vi "Galvo+Histo.vi"() -> ()   [LabVIEW 2016]
uses:
  <vilib>/Utility/error.llb/DialogType.ctl
  <vilib>/DAQmx/write.llb/DAQmx Write (Analog 1D DBL NChan 1Samp).vi
  <vilib>/DAQmx/write.llb/DAQmx Write (Analog DBL 1Chan 1Samp).vi
  <vilib>/DAQmx/create/channels.llb/DAQmx Create Channel (AO-Voltage-Basic).vi
  <vilib>/DAQmx/miscellaneous.llb/DAQmx Fill In Error Info.vi
  HHLib64.dll
panel:
  in  "Run":bool
  in  "done":bool
  in  "Syncdiv":enum16{"1", "2", "4", "8"}(ring)
  in  "Binning":i32 min=0 max=10 step=1
  in  "Sync Level":i32=50 min=0 max=800 step=10
  in  "Ch1 Level":i32=50 min=0 max=800 step=10
  in  "Ch1 ZeroX":i32=10 min=0 max=20 step=1
  in  "Sync ZeroX":i32=10 min=0 max=20 step=1
  in  "Sync Offs":i32=-10000 min=-99999 max=99999 step=1
  in  "Ch1 Offs":i32 min=-99999 max=99999 step=1
  in  "Ch2 Level":i32=50 min=0 max=800 step=10
  in  "Ch2 ZeroX":i32=10 min=0 max=20 step=1
  in  "Ch2 Offs":i32 min=-99999 max=99999 step=1
  in  "Ch3 Level":i32=50 min=0 max=800 step=10
  in  "Ch3 ZeroX":i32=10 min=0 max=20 step=1
  in  "Ch3 Offs":i32 min=-99999 max=99999 step=1
  in  "Ch4 Offs":i32 min=-99999 max=99999 step=1
  in  "Ch4 Level":i32=50 min=0 max=800 step=10
  in  "Ch4 ZeroX":i32=10 min=0 max=20 step=1
  out "Resol / ps":dbl format="%.2f"
  in  "Ch8 ZeroX":i32=10 min=0 max=20 step=1
  in  "Ch8 Level":i32=50 min=0 max=800 step=10
  in  "Ch8 Offs":i32 min=-99999 max=99999 step=1
  in  "Ch7 Offs":i32 min=-99999 max=99999 step=1
  in  "Ch7 ZeroX":i32=10 min=0 max=20 step=1
  in  "Ch7 Level":i32=50 min=0 max=800 step=10
  in  "Ch5 Level":i32=50 min=0 max=800 step=10
  in  "Ch6 Level":i32=50 min=0 max=800 step=10
  in  "Ch5 ZeroX":i32=10 min=0 max=20 step=1
  in  "Ch6 ZeroX":i32=10 min=0 max=20 step=1
  in  "Ch5 Offs":i32 min=-99999 max=99999 step=1
  in  "Ch6 Offs":i32 min=-99999 max=99999 step=1
  out "Oveflow":bool
  out "Histogram":u32[][](graph)
  out "IntegralCount":i32[](array[numeric])
  in  "Acq.Time /ms":i32=1000 min=1 max=3600000 step=100
  out "Rate 4":i32(slide) scale=0.01..100000000.0 scale format="%.0e"
  out "Rate 3":i32(slide) scale=0.01..100000000.0 scale format="%.0e"
  out "Rate 2":i32(slide) scale=0.01..100000000.0 scale format="%.0e"
  out "Rate 1":i32(slide) scale=0.01..100000000.0 scale format="%.0e"
  out "Sync Rate":i32(slide) scale=0.01..100000000.0 scale format="%.0e"
  out "Rate 6":i32(slide) scale=0.01..100000000.0 scale format="%.0e"
  out "Rate 5":i32(slide) scale=0.01..100000000.0 scale format="%.0e"
  out "Rate 7":i32(slide) scale=0.01..100000000.0 scale format="%.0e"
  out "Rate 8":i32(slide) scale=0.01..100000000.0 scale format="%.0e"
  out "Warnings":string
  out "Serial Num.":string
  out "DeviceIndex":i32=-1
  out "DLL Version (must be 2.0)":string caption="DLL Version"
  out "Calibration Status":string
  out "Initialization Status":string
  in  "Hold/Scan":enum32{"Hold", "Radio Selection 2"}(radio)
  in  "Max Voltage":dbl=10.0
  in  "Min Voltage Voltage":dbl=-10.0
  in  "Set this opposite to one above":tag="Dev1/ao0"
  out "Current Voltage":dbl
  out "Next Voltage":dbl
  in  "Wait Time (ms)":dbl=100.0
  in  "Max Voltage 2":dbl=10.0
  in  "Min Voltage Voltage 2":dbl=-10.0
  in  "Scan in X: Set to ao1\nScan in Y: Set to ao0":tag="Dev1/ao0"
  out "Current Voltage 2":dbl
  out "Next Voltage 2":dbl
  in  "Wait Time (ms) 2":dbl=100.0
  in  "Voltage Step 2":dbl=0.1
  in  "Voltage Step":dbl=0.1
  in  "Physical Channel(s)":tag="Dev1/ao0"
  in  "Stop":bool
  in  "Output Voltage":dbl[](array[numeric])
  in  "Min Voltage":dbl=-10.0
  in  "Max Voltage 3":dbl=10.0
  in  "Physical Channel(s)  2":tag="Dev1/ao0"
  in  "Stop 2":bool
  in  "Output Voltage 2":dbl[](array[numeric])
  in  "Min Voltage 2":dbl=-10.0
  in  "Max Voltage 4":dbl=10.0
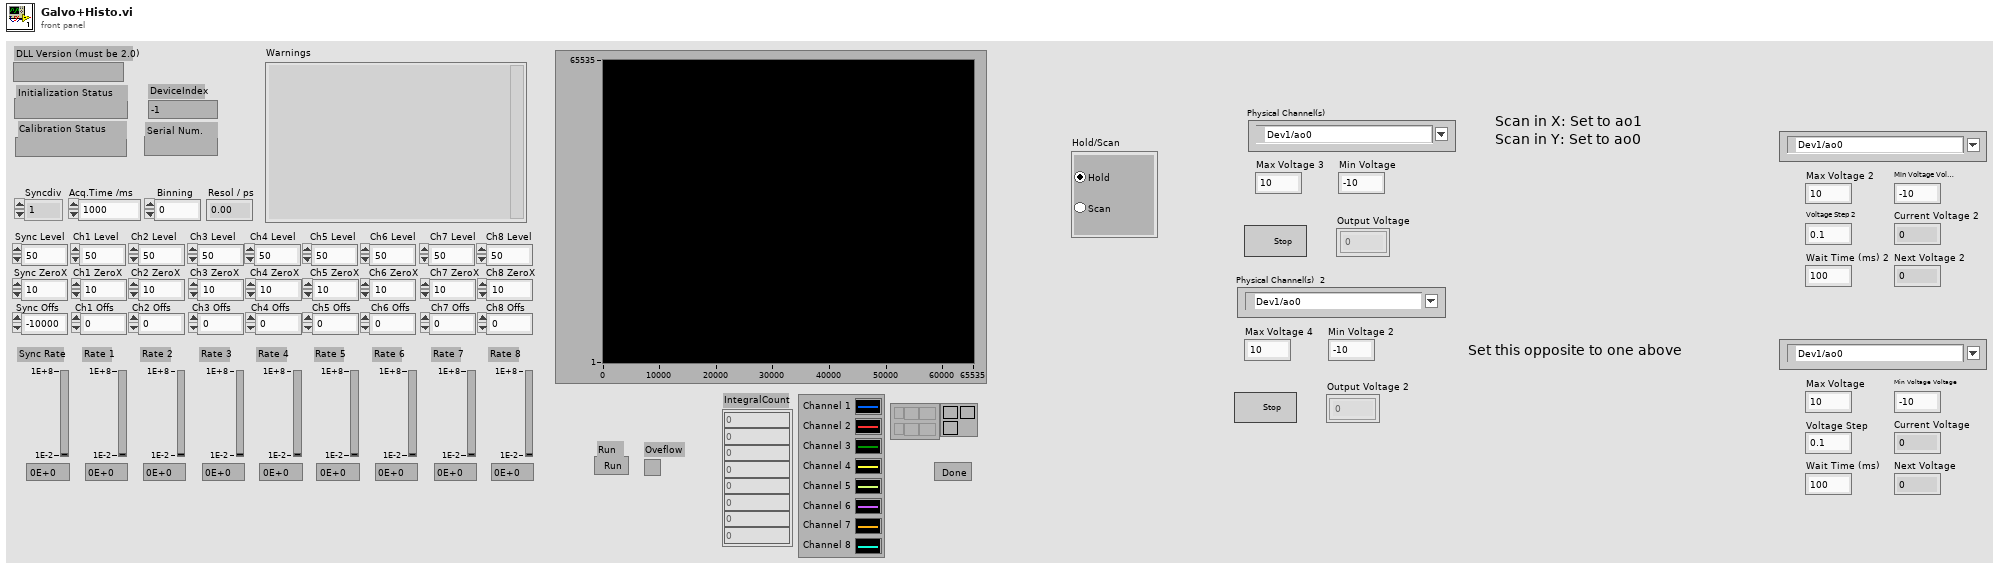
[diagram p1: front panel]
types:
  T1 = cluster{"rate":i32, "rate":i32, "rate":i32, "rate":i32, "rate":i32, "rate":i32, "rate":i32, "rate":i32}
  T2 = typedef "DialogType.ctl" = u16
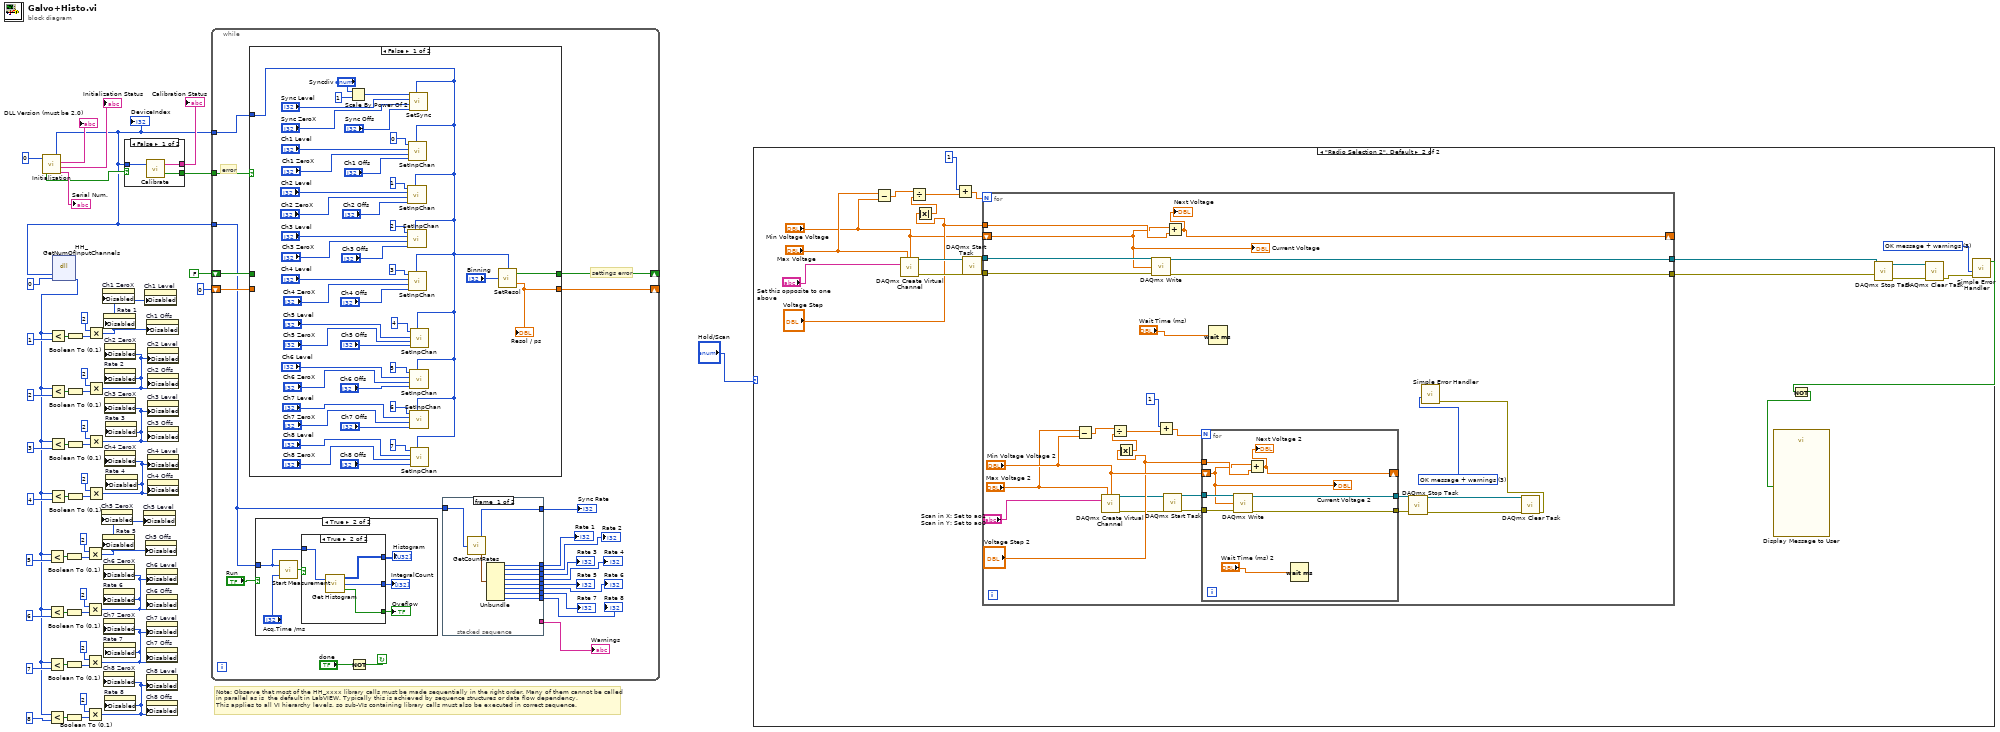
[diagram p0: block diagram]
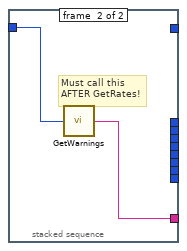
[diagram p2: hidden frame]
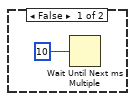
[diagram p3: hidden frame]
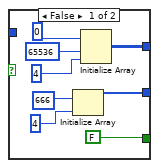
[diagram p4: hidden frame]
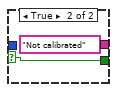
[diagram p6: hidden frame]
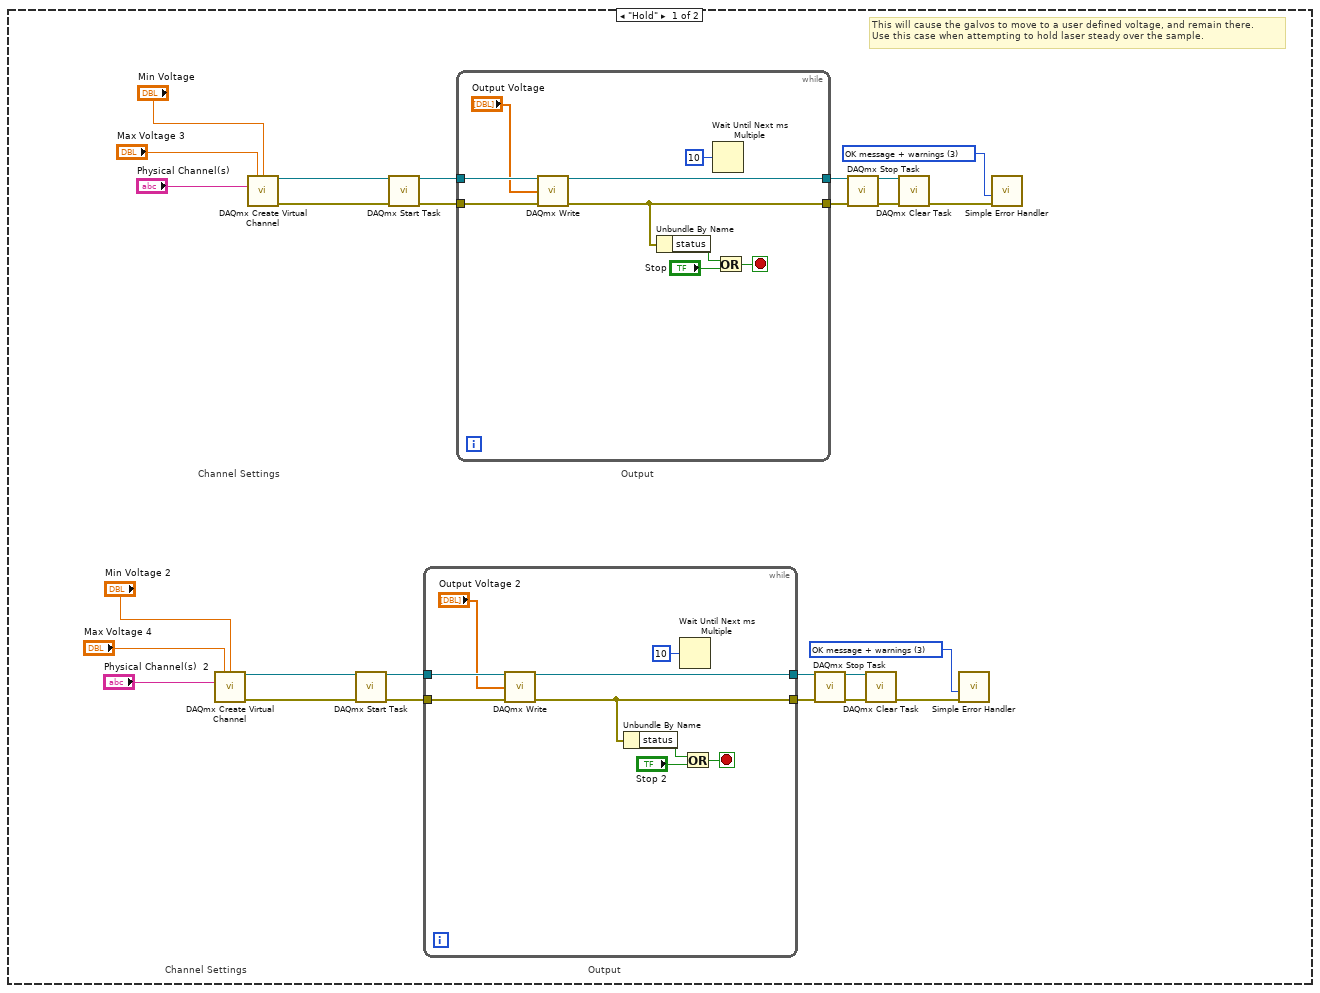
[diagram p7: hidden frame]
diagram:
  # "settings error"
  # "Note: Observe that most of the HH_xxxx library calls must be made sequentially in the right order. Many of them cannot be called \nin parallel as is  the default in LabVIEW. Typically this is achieved by sequence structures or data flow dependency. \nThis applies to all VI hierarchy levels, so sub-VIs containing library calls must also be executed in correct sequence."
  n1 = call "Initialization.vi"("Mode"=0) -> ("Initialisation Error"=w45:bool, "Deviceindex"=w23:i32, "DLL Version"=→"DLL Version (must be 2.0)":string, "Initialization Status"=→"Initialization Status":string, "Serial[8]"=→"Serial Num.":string)
  "DeviceIndex" <- w23
  n2 = dll-call lib="HHLib64.dll" fn="HH_GetNumOfInputChannels" label="HH_GetNumOfCh"("devidx"=w23, "numch"=0) -> ("numch"=w1:i32)  [unwired: 5 in, 2 out]
  n3 = Less?(x=w1, y=5) -> (x < y?=w20:bool)
  n4 = Less?(x=w1, y=6) -> (x < y?=w15:bool)
  n5 = Less?(x=w1, y=7) -> (x < y?=w11:bool)
  n6 = Less?(x=w1, y=8) -> (x < y?=w7:bool)
  n7 = Less?(x=w1, y=1) -> (x < y?=w42:bool)
  n8 = Less?(x=w1, y=2) -> (x < y?=w37:bool)
  n9 = Less?(x=w1, y=3) -> (x < y?=w33:bool)
  n10 = Less?(x=w1, y=4) -> (x < y?=w29:bool)
  n11 = Boolean To (0,1)(Boolean=w20) -> (0, 1=w19:i16)
  n12 = Boolean To (0,1)(Boolean=w15) -> (0, 1=w16:i16)
  n13 = Boolean To (0,1)(Boolean=w11) -> (0, 1=w12:i16)
  n14 = Boolean To (0,1)(Boolean=w7) -> (0, 1=w8:i16)
  n15 = Boolean To (0,1)(Boolean=w42) -> (0, 1=w41:i16)
  n16 = Boolean To (0,1)(Boolean=w37) -> (0, 1=w38:i16)
  n17 = Boolean To (0,1)(Boolean=w33) -> (0, 1=w34:i16)
  n18 = Boolean To (0,1)(Boolean=w29) -> (0, 1=w30:i16)
  n19 = Multiply(x=2, y=w19) -> (x*y=w2:i32)
  n20 = Multiply(x=2, y=w16) -> (x*y=w3:i32)
  n21 = Multiply(x=2, y=w12) -> (x*y=w4:i32)
  n22 = Multiply(x=2, y=w8) -> (x*y=w5:i32)
  n23 = Multiply(x=2, y=w41) -> (x*y=w24:i32)
  n24 = Multiply(x=2, y=w38) -> (x*y=w25:i32)
  n25 = Multiply(x=2, y=w34) -> (x*y=w26:i32)
  n26 = Multiply(x=2, y=w30) -> (x*y=w27:i32)
  n27 = property on="Ch5 ZeroX" class="DigNum (strict)"("Disabled"=w2) -> ()  [unwired: 2 in, 2 out]
  n28 = property on="Ch1 ZeroX" class="DigNum (strict)"("Disabled"=w24) -> ()  [unwired: 2 in, 2 out]
  n29 = property on="Rate 5" class="Slide (strict)"("Disabled"=w2) -> ()  [unwired: 2 in, 2 out]
  n30 = property on="Ch6 ZeroX" class="DigNum (strict)"("Disabled"=w3) -> ()  [unwired: 2 in, 2 out]
  n31 = property on="Rate 6" class="Slide (strict)"("Disabled"=w3) -> ()  [unwired: 2 in, 2 out]
  n32 = property on="Ch7 ZeroX" class="DigNum (strict)"("Disabled"=w4) -> ()  [unwired: 2 in, 2 out]
  n33 = property on="Ch8 ZeroX" class="DigNum (strict)"("Disabled"=w5) -> ()  [unwired: 2 in, 2 out]
  n34 = property on="Rate 1" class="Slide (strict)"("Disabled"=w24) -> ()  [unwired: 2 in, 2 out]
  n35 = property on="Rate 7" class="Slide (strict)"("Disabled"=w4) -> ()  [unwired: 2 in, 2 out]
  n36 = property on="Ch2 ZeroX" class="DigNum (strict)"("Disabled"=w25) -> ()  [unwired: 2 in, 2 out]
  n37 = property on="Rate 2" class="Slide (strict)"("Disabled"=w25) -> ()  [unwired: 2 in, 2 out]
  n38 = property on="Ch3 ZeroX" class="DigNum (strict)"("Disabled"=w26) -> ()  [unwired: 2 in, 2 out]
  n39 = property on="Ch4 ZeroX" class="DigNum (strict)"("Disabled"=w27) -> ()  [unwired: 2 in, 2 out]
  n40 = property on="Rate 8" class="Slide (strict)"("Disabled"=w5) -> ()  [unwired: 2 in, 2 out]
  n41 = property on="Rate 3" class="Slide (strict)"("Disabled"=w26) -> ()  [unwired: 2 in, 2 out]
  n42 = property on="Rate 4" class="Slide (strict)"("Disabled"=w27) -> ()  [unwired: 2 in, 2 out]
  n43 = case shown="False" w45 {
    selector: w45 -> [_ w57]
    tunnel: [w56 "Not calibrated"] -> w52
    tunnel: [w55 w57] -> w50
    tunnel: w23 -> [w54 _]
    frame False {
      n44 = call "Calibrate.vi"("Deviceindex"=w54) -> ("Calib Error"=w55:bool, "Status"=w56:string)  [unwired: 1 in]
    }
    frame True {
    }
  }
  "Calibration Status" <- w52
  n45 = property on="Ch5 Level" class="DigNum (strict)"("Disabled"=w2) -> ()  [unwired: 2 in, 2 out]
  n46 = property on="Ch1 Level" class="DigNum (strict)"("Disabled"=w24) -> ()  [unwired: 2 in, 2 out]
  n47 = property on="Ch5 Offs" class="DigNum (strict)"("Disabled"=w2) -> ()  [unwired: 2 in, 2 out]
  n48 = property on="Ch6 Level" class="DigNum (strict)"("Disabled"=w3) -> ()  [unwired: 2 in, 2 out]
  n49 = property on="Ch6 Offs" class="DigNum (strict)"("Disabled"=w3) -> ()  [unwired: 2 in, 2 out]
  n50 = property on="Ch7 Level" class="DigNum (strict)"("Disabled"=w4) -> ()  [unwired: 2 in, 2 out]
  n51 = property on="Ch7 Offs" class="DigNum (strict)"("Disabled"=w4) -> ()  [unwired: 2 in, 2 out]
  n52 = property on="Ch8 Level" class="DigNum (strict)"("Disabled"=w5) -> ()  [unwired: 2 in, 2 out]
  n53 = property on="Ch8 Offs" class="DigNum (strict)"("Disabled"=w5) -> ()  [unwired: 2 in, 2 out]
  n54 = property on="Ch1 Offs" class="DigNum (strict)"("Disabled"=w24) -> ()  [unwired: 2 in, 2 out]
  n55 = property on="Ch2 Level" class="DigNum (strict)"("Disabled"=w25) -> ()  [unwired: 2 in, 2 out]
  n56 = property on="Ch2 Offs" class="DigNum (strict)"("Disabled"=w25) -> ()  [unwired: 2 in, 2 out]
  n57 = property on="Ch3 Level" class="DigNum (strict)"("Disabled"=w26) -> ()  [unwired: 2 in, 2 out]
  n58 = property on="Ch3 Offs" class="DigNum (strict)"("Disabled"=w26) -> ()  [unwired: 2 in, 2 out]
  n59 = property on="Ch4 Level" class="DigNum (strict)"("Disabled"=w27) -> ()  [unwired: 2 in, 2 out]
  n60 = property on="Ch4 Offs" class="DigNum (strict)"("Disabled"=w27) -> ()  [unwired: 2 in, 2 out]
  n61 = while {
    tunnel: w23 -> [w69]
    tunnel: w23 -> [w70]
    tunnel: w50 -> [w74]
    shift-left: 0 -> [w75]
    shift-right: [w76] -> _
    shift-left: FALSE -> [w73]
    shift-right: [w71] -> _
    stop <- w77 continue-if-true
    # "error"
    n62 = case shown="False" w74 {
      tunnel: [w129 w154] -> w71
      tunnel: w73 -> [_ w154]
      tunnel: [w128 w153] -> w76
      tunnel: w75 -> [_ w153]
      tunnel: w70 -> [w111 _]
      frame False {
        n63 = Scale By Power Of 2(n="Syncdiv", x=1) -> (x*2^n=w150:i32)
        n64 = call "SetInpChan.vi"("Channel"=1, "CFD Level"="Ch2 Level", "CFD ZeroX"="Ch2 ZeroX", "Offset"="Ch2 Offs", "DeviceIndex"=w111) -> ()  [unwired: 1 in, 1 out]
        n65 = call "SetInpChan.vi"("Channel"=2, "CFD Level"="Ch3 Level", "CFD ZeroX"="Ch3 ZeroX", "Offset"="Ch3 Offs", "DeviceIndex"=w111) -> ()  [unwired: 1 in, 1 out]
        n66 = call "SetInpChan.vi"("Channel"=0, "CFD Level"="Ch1 Level", "CFD ZeroX"="Ch1 ZeroX", "Offset"="Ch1 Offs", "DeviceIndex"=w111) -> ()  [unwired: 1 in, 1 out]
        n67 = call "SetInpChan.vi"("Channel"=3, "CFD Level"="Ch4 Level", "CFD ZeroX"="Ch4 ZeroX", "Offset"="Ch4 Offs", "DeviceIndex"=w111) -> ()  [unwired: 1 in, 1 out]
        n68 = call "SetSync.vi"("SyncDiv"=w150, "CFD Level"="Sync Level", "CFD ZeroX"="Sync ZeroX", "Offset"="Sync Offs", "DeviceIndex"=w111) -> ()  [unwired: 1 in, 1 out]
        n69 = call "SetInpChan.vi"("Channel"=5, "CFD Level"="Ch6 Level", "CFD ZeroX"="Ch6 ZeroX", "Offset"="Ch6 Offs", "DeviceIndex"=w111) -> ()  [unwired: 1 in, 1 out]
        n70 = call "SetInpChan.vi"("Channel"=6, "CFD Level"="Ch7 Level", "CFD ZeroX"="Ch7 ZeroX", "Offset"="Ch7 Offs", "DeviceIndex"=w111) -> ()  [unwired: 1 in, 1 out]
        n71 = call "SetInpChan.vi"("Channel"=4, "CFD Level"="Ch5 Level", "CFD ZeroX"="Ch5 ZeroX", "Offset"="Ch5 Offs", "DeviceIndex"=w111) -> ()  [unwired: 1 in, 1 out]
        n72 = call "SetInpChan.vi"("Channel"=7, "CFD Level"="Ch8 Level", "CFD ZeroX"="Ch8 ZeroX", "Offset"="Ch8 Offs", "DeviceIndex"=w111) -> ()  [unwired: 1 in, 1 out]
        n73 = call "SetResol.vi"("DeviceIndex"=w111, "Binning"="Binning") -> ("Resolution"=w128:dbl, "Error"=w129:bool)  [unwired: 2 in]
        "Resol / ps" <- w128
      }
      frame True {
      }
    }
    n74 = case shown="True" "Run" {
      tunnel: w69 -> [_ w94]
      frame False {
        n75 = Wait Until Next ms Multiple(millisecond multiple=10) -> ()  [unwired: 1 out]
      }
      frame True {
        n76 = call "Start Measurement.vi"("Acquisition time"="Acq.Time /ms", "DeviceIndex"=w94) -> ("DataValid"=w98:bool)
        n77 = case shown="True" w98 {
          tunnel: [FALSE w110] -> w97
          tunnel: [w100 w109] -> w96
          tunnel: [w99 w108] -> w95
          tunnel: w94 -> [_ w107]
          frame False {
            n78 = Initialize Array(u32 666, 4) -> (w99:u32[])
            n79 = Initialize Array(u32 0, 65536, 4) -> (w100:u32[][])
          }
          frame True {
            n80 = call "Get Histogram.vi"("DeviceIndex"=w107) -> ("Histograms"=w109:u32[][], "IntegralCount"=w108:i32[], "Overflow"=w110:bool)  [unwired: 1 in]
          }
        }
        "Oveflow" <- w97
        "Histogram" <- w96
        "IntegralCount" <- w95
      }
    }
    n81 = Not(x="done") -> (.not. x?=w77:bool)
    n82 = stacked-sequence {
      tunnel: w69 -> [w89 w90]
      tunnel: [w88 _] -> w68
      tunnel: [w86 _] -> w67
      tunnel: [w85 _] -> w66
      tunnel: [w84 _] -> w65
      tunnel: [w83 _] -> w64
      tunnel: [w82 _] -> w63
      tunnel: [w81 _] -> w62
      tunnel: [w80 _] -> w61
      tunnel: [w79 _] -> w60
      tunnel: [_ w91] -> w59
      frame #0 {
        n83 = call "GetCountRates.vi"("DeviceIndex"=w89) -> ("SyncRate"=w88:i32, "Count Rates"=w87:T1)
        n84 = Unbundle(w87) -> ("rate"=w86:i32, "rate"=w85:i32, "rate"=w84:i32, "rate"=w83:i32, "rate"=w82:i32, "rate"=w81:i32, "rate"=w80:i32, "rate"=w79:i32)
      }
      frame #1 {
        # "Must call this\nAFTER GetRates!"
        n85 = call "GetWarnings.vi"("Deviceindex"=w90) -> ("warningstext"=w91:string)
      }
    }
    "Rate 4" <- w64
    "Rate 3" <- w65
    "Rate 2" <- w66
    "Rate 1" <- w67
    "Sync Rate" <- w68
    "Rate 6" <- w62
    "Rate 5" <- w63
    "Rate 7" <- w61
    "Rate 8" <- w60
    "Warnings" <- w59
  }
  n86 = case shown="\"Radio Selection 2\", Default" "Hold/Scan" {
    frame "Hold" {
      w157 = T2 3 items=["no dialog", "OK message", "continue or stop message", "OK message + warnings", "continue/stop + warnings"] ("type of dialog (OK msg:1)")
      w170 = T2 3 items=["no dialog", "OK message", "continue or stop message", "OK message + warnings", "continue/stop + warnings"] ("type of dialog (OK msg:1)")
      # "Output"
      # "Channel Settings"
      # "This will cause the galvos to move to a user defined voltage, and remain there.\nUse this case when attempting to hold laser steady over the sample."
      # "Output"
      # "Channel Settings"
      n87 = call-poly <vilib>:"DAQmx Create Virtual Channel.vi"("maximum value"="Max Voltage 4", "minimum value"="Min Voltage 2", "physical channels"="Physical Channel(s)  2") -> ("task out"=w165:refnum<k21>, "error out"=w164:errorcluster)  [unwired: 11 in]
      n88 = call-poly <vilib>:"DAQmx Create Virtual Channel.vi"("maximum value"="Max Voltage 3", "minimum value"="Min Voltage", "physical channels"="Physical Channel(s)") -> ("task out"=w178:refnum<k21>, "error out"=w177:errorcluster)  [unwired: 11 in]
      n89 = call <vilib>:"DAQmx Start Task.vi"("task/channels in"=w165, "error in"=w164) -> ("task out"=w163:refnum<k21>, "error out"=w162:errorcluster)  [unwired: 12 in]
      n90 = call <vilib>:"DAQmx Start Task.vi"("task/channels in"=w178, "error in"=w177) -> ("task out"=w176:refnum<k21>, "error out"=w175:errorcluster)  [unwired: 12 in]
      n91 = while {
        tunnel: w163 -> [w189]
        tunnel: w162 -> [w188]
        tunnel: [w183] -> w160
        tunnel: [w187] -> w161
        stop <- w181 stop-if-true
        n92 = call-poly <vilib>:"DAQmx Write.vi"("task/channels in"=w189, "data"="Output Voltage 2", "error in"=w188) -> ("task out"=w187:refnum<k21>, "error out"=w183:errorcluster)  [unwired: 10 in, 1 out]
        n93 = Unbundle By Name(w183) -> ("status"=w185:bool)
        n94 = Wait Until Next ms Multiple(millisecond multiple=u32 10) -> ()  [unwired: 1 out]
        n95 = Or(x=w185, y="Stop 2") -> (x .or. y?=w181:bool)
      }
      n96 = while {
        tunnel: w176 -> [w198]
        tunnel: w175 -> [w197]
        tunnel: [w192] -> w173
        tunnel: [w196] -> w174
        stop <- w190 stop-if-true
        n97 = call-poly <vilib>:"DAQmx Write.vi"("task/channels in"=w198, "data"="Output Voltage", "error in"=w197) -> ("task out"=w196:refnum<k21>, "error out"=w192:errorcluster)  [unwired: 10 in, 1 out]
        n98 = Unbundle By Name(w192) -> ("status"=w194:bool)
        n99 = Wait Until Next ms Multiple(millisecond multiple=u32 10) -> ()  [unwired: 1 out]
        n100 = Or(x=w194, y="Stop") -> (x .or. y?=w190:bool)
      }
      n101 = call <vilib>:"DAQmx Stop Task.vi"("task/channels in"=w161, "error in"=w160) -> ("task out"=w159:refnum<k21>, "error out"=w158:errorcluster)  [unwired: 12 in]
      n102 = call <vilib>:"DAQmx Stop Task.vi"("task/channels in"=w174, "error in"=w173) -> ("task out"=w172:refnum<k21>, "error out"=w171:errorcluster)  [unwired: 12 in]
      n103 = call <vilib>:"DAQmx Clear Task.vi"("task in"=w159, "error in"=w158) -> ("error out"=w167:errorcluster)  [unwired: 13 in]
      n104 = call <vilib>:"DAQmx Clear Task.vi"("task in"=w172, "error in"=w171) -> ("error out"=w180:errorcluster)  [unwired: 13 in]
      n105 = call <vilib>:"Simple Error Handler.vi"("type of dialog (OK msg:1)"=w157, "error in (no error)"=w167) -> ()  [unwired: 3 in, 5 out]
      n106 = call <vilib>:"Simple Error Handler.vi"("type of dialog (OK msg:1)"=w170, "error in (no error)"=w180) -> ()  [unwired: 3 in, 5 out]
    }
    frame "Radio Selection 2", Default {
      w210 = T2 3 items=["no dialog", "OK message", "continue or stop message", "OK message + warnings", "continue/stop + warnings"] ("type of dialog (OK msg:1)")
      n107 = Subtract(x="Max Voltage", y="Min Voltage Voltage") -> (x-y=w207:dbl)
      n108 = call-poly <vilib>:"DAQmx Create Virtual Channel.vi"("maximum value"="Max Voltage", "minimum value"="Min Voltage Voltage", "physical channels"="Set this opposite to one above") -> ("task out"=w218:refnum<k21>, "error out"=w217:errorcluster)  [unwired: 11 in]
      n109 = Absolute Value(x="Voltage Step") -> (abs(x)=w205:dbl)
      n110 = Divide(x=w207, y=w205) -> (x/y=w203:dbl)
      n111 = Add(x=1, y=w203) -> (x+y=w201:dbl)
      n112 = call <vilib>:"DAQmx Start Task.vi"("task/channels in"=w218, "error in"=w217) -> ("task out"=w216:refnum<k21>, "error out"=w215:errorcluster)  [unwired: 12 in]
      n113 = for {
        N: w201 -> [_]
        tunnel: w216 -> [w246]
        tunnel: w215 -> [w245]
        tunnel: [w244] -> w214
        tunnel: [w242] -> w213
        tunnel: "Voltage Step" -> [w243]
        shift-right: [w240] -> _
        shift-left: "Min Voltage Voltage" -> [w241]
        w230 = T2 3 items=["no dialog", "OK message", "continue or stop message", "OK message + warnings", "continue/stop + warnings"] ("type of dialog (OK msg:1)")
        n114 = Subtract(x="Max Voltage 2", y="Min Voltage Voltage 2") -> (x-y=w233:dbl)
        n115 = call-poly <vilib>:"DAQmx Create Virtual Channel.vi"("maximum value"="Max Voltage 2", "minimum value"="Min Voltage Voltage 2", "physical channels"="Scan in X: Set to ao1\nScan in Y: Set to ao0") -> ("task out"=w222:refnum<k21>, "error out"=w223:errorcluster)  [unwired: 11 in]
        n116 = Absolute Value(x="Voltage Step 2") -> (abs(x)=w235:dbl)
        n117 = Divide(x=w233, y=w235) -> (x/y=w237:dbl)
        n118 = call-poly <vilib>:"DAQmx Write.vi"("task/channels in"=w246, "data"=w241, "error in"=w245) -> ("task out"=w242:refnum<k21>, "error out"=w244:errorcluster)  [unwired: 10 in, 1 out]
        n119 = Add(x=1, y=w237) -> (x+y=w238:dbl)
        n120 = call <vilib>:"DAQmx Start Task.vi"("task/channels in"=w222, "error in"=w223) -> ("task out"=w224:refnum<k21>, "error out"=w225:errorcluster)  [unwired: 12 in]
        n121 = Add(x=w241, y=w243) -> (x+y=w240:dbl)
        "Next Voltage" <- w240
        n122 = for {
          N: w238 -> [_]
          tunnel: w224 -> [w254]
          tunnel: w225 -> [w253]
          tunnel: [w252] -> w226
          tunnel: [w250] -> w227
          tunnel: "Voltage Step 2" -> [w251]
          shift-right: [w248] -> _
          shift-left: "Min Voltage Voltage 2" -> [w249]
          n123 = call-poly <vilib>:"DAQmx Write.vi"("task/channels in"=w254, "data"=w249, "error in"=w253) -> ("task out"=w250:refnum<k21>, "error out"=w252:errorcluster)  [unwired: 10 in, 1 out]
          n124 = Add(x=w249, y=w251) -> (x+y=w248:dbl)
          "Next Voltage 2" <- w248
          n125 = Wait (ms)(milliseconds to wait="Wait Time (ms) 2") -> ()  [unwired: 1 out]
          "Current Voltage 2" <- w249
        }
        n126 = Wait (ms)(milliseconds to wait="Wait Time (ms)") -> ()  [unwired: 1 out]
        n127 = call <vilib>:"DAQmx Stop Task.vi"("task/channels in"=w227, "error in"=w226) -> ("task out"=w229:refnum<k21>, "error out"=w228:errorcluster)  [unwired: 12 in]
        n128 = call <vilib>:"DAQmx Clear Task.vi"("task in"=w229, "error in"=w228) -> ("error out"=w231:errorcluster)  [unwired: 13 in]
        n129 = call <vilib>:"Simple Error Handler.vi"("type of dialog (OK msg:1)"=w230, "error in (no error)"=w231) -> ()  [unwired: 3 in, 5 out]
        "Current Voltage" <- w241
      }
      n130 = call <vilib>:"DAQmx Stop Task.vi"("task/channels in"=w213, "error in"=w214) -> ("task out"=w211:refnum<k21>, "error out"=w212:errorcluster)  [unwired: 12 in]
      n131 = call <vilib>:"DAQmx Clear Task.vi"("task in"=w211, "error in"=w212) -> ("error out"=w209:errorcluster)  [unwired: 13 in]
      n132 = call <vilib>:"Simple Error Handler.vi"("type of dialog (OK msg:1)"=w210, "error in (no error)"=w209) -> ("error?"=w200:bool)  [unwired: 3 in, 4 out]
      n133 = Not(x=w200) -> (.not. x?=w199:bool)
      n134 = call "Display Message to User"("Enable"=w199) -> ()  [unwired: 9 in, 2 out]
    }
  }
